vi "send_to_main_queue.vi"(8 "error in (no error)":errorcluster, 11 "Main_state_cluster":T1) -> (0 "error out":errorcluster)   [LabVIEW 2011, in "Fiberscope_library.lvlib"]
uses:
  Fiberscope_library.lvlib
  typedefs/main_state_cluster.ctl
  typedefs/main_state_enum.ctl
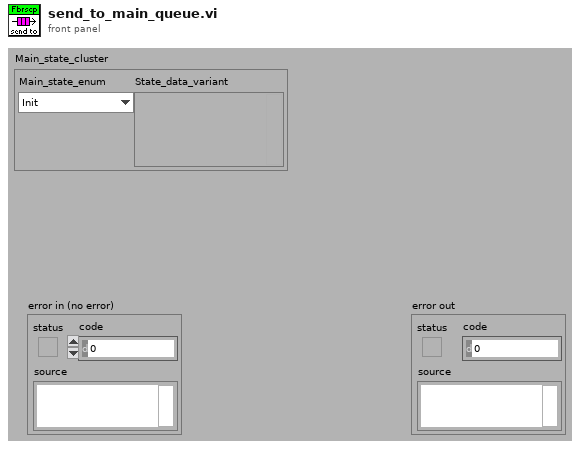
[diagram p1: front panel]
types:
  T1 = typedef "Fiberscope_library.lvlib/main_state_cluster.ctl" = cluster{"Main_state_enum":T2, "State_data_variant":variant}
  T2 = typedef "Fiberscope_library.lvlib/main_state_enum.ctl" = enum16{"Init", "Error", "Quit", "Run_cont", "Stop", "Change_parameters", "Timeout", "Shutter", "Run_noframes", "Save", "Wait_for_finished", "Change_storage", "Change_pixelmap", "Change_averages"}
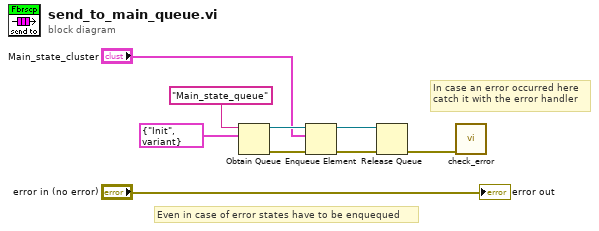
[diagram p0: block diagram]
diagram:
  # "In case an error occurred here\ncatch it with the error handler"
  # "Even in case of error states have to be enquequed"
  n1 = Obtain Queue(name (unnamed)="Main_state_queue", element data type=T1 {"Main_state_enum"=enum."Init", "State_data_variant"=variant} ("Main_state_cluster")) -> (queue out=w7:refnum<queue>, error out=w8:errorcluster)  [unwired: 3 in, 1 out]
  n2 = Enqueue Element(queue=w7, element="Main_state_cluster", error in (no error)=w8) -> (queue out=w3:refnum<queue>, error out=w2:errorcluster)  [unwired: 1 in, 1 out]
  n3 = Release Queue(queue=w3, error in (no error)=w2) -> (error out=w1:errorcluster)  [unwired: 1 in, 2 out]
  n4 = call "check_error.vi"("error in"=w1) -> ()  [unwired: 10 in, 1 out]
  "error out" <- "error in (no error)"
